vi "WM_CAP - Get Camera Name.vi"(11 "error in (no error)":errorcluster) -> (6 "FriendlyName":string, 8 "Connected?":bool, 15 "error out":errorcluster)   [LabVIEW 2022 SP3]
uses:
  <vilib>/registry/registry.llb/Registry RtKey.ctl
  <vilib>/registry/registry.llb/Read Registry Value Simple STR.vi
  <vilib>/registry/registry.llb/Read Registry Value Simple U32.vi
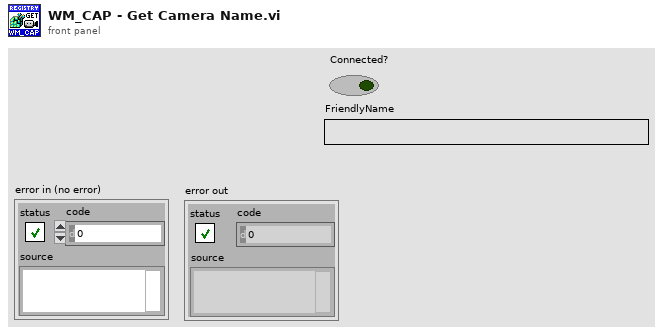
[diagram p1: front panel]
types:
  T1 = typedef "Registry RtKey.ctl" = enum32{"HKEY_CLASSES_ROOT", "HKEY_CURRENT_USER", "HKEY_LOCAL_MACHINE", "HKEY_USERS", "HKEY_PERFORMANCE_DATA", "HKEY_CURRENT_CONFIG", "HKEY_DYN_DATA"}
  T2 = typedef "Registry refnum.ctl" = refnum<k1>
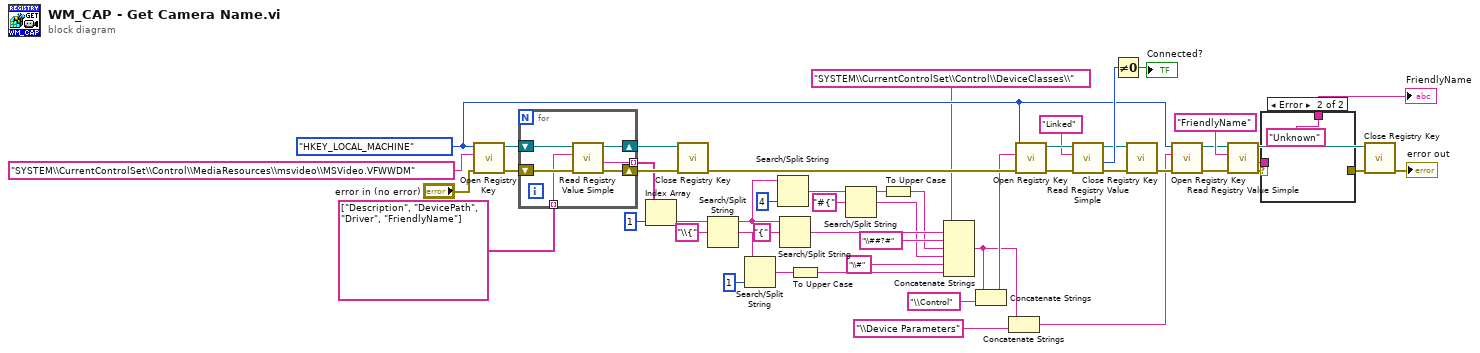
[diagram p0: block diagram]
diagram:
  w10 = Registry_RtKey."HKEY_LOCAL_MACHINE" ("root key (HKEY_LOCAL_MACHINE)")
  n1 = call <vilib>:"Open Registry Key.vi"("error in (no error)"="error in (no error)", "subkey"="SYSTEM\\CurrentControlSet\\Control\\MediaResources\\msvideo\\MSVideo.VFWWDM", "root key (HKEY_LOCAL_MACHINE)"=w10) -> ("error out"=w46:errorcluster, "refnum out"=w47:T2)  [unwired: 7 in]
  n2 = for {
    shift-right: [w55] -> w50
    shift-left: w47 -> [w57]
    shift-right: [w54] -> w49
    shift-left: w46 -> [w56]
    tunnel: string[] ["Description", "DevicePath", "Driver", "FriendlyName"] -> [w53] mode=indexing
    tunnel: [w52] -> w45 mode=indexing
    n3 = call-poly <vilib>:"Read Registry Value Simple.vi"("error in (no error)"=w56, "value"=w53, "refnum"=w57) -> ("error out"=w54:errorcluster, "String/Binary data"=w52:string, "refnum out"=w55:T2)  [unwired: 3 in, 1 out]
  }
  n4 = Index Array(array=w45, index=1) -> (element=w38:string)
  n5 = call <vilib>:"Close Registry Key.vi"("error in (no error)"=w49, "refnum"=w50) -> ("error out"=w39:errorcluster)  [unwired: 5 in]
  n6 = Search/Split String(string=w38, search string/char (-)="\\{") -> (substring before match=w35:string, match + rest of string=w41:string)  [unwired: 1 in, 1 out]
  n7 = Search/Split String(string=w41, offset (0)=1) -> (match + rest of string=w33:string)  [unwired: 1 in, 2 out]
  n8 = Search/Split String(string=w35, offset (0)=4) -> (match + rest of string=w27:string)  [unwired: 1 in, 2 out]
  n9 = Search/Split String(string=w35, search string/char (-)="{") -> (match + rest of string=w37:string)  [unwired: 1 in, 2 out]
  n10 = To Upper Case(1:w33) -> (0:w31:string)
  n11 = Search/Split String(string=w27, search string/char (-)="#{") -> (substring before match=w25:string, match + rest of string=w23:string)  [unwired: 1 in, 1 out]
  n12 = To Upper Case(1:w25) -> (0:w24:string)
  n13 = Concatenate Strings("SYSTEM\\CurrentControlSet\\Control\\DeviceClasses\\" ("subkey"), w37, "\\##?#" ("string"), w24, w23, "\\#" ("string"), w31) -> (w18:string)
  n14 = Concatenate Strings(w18, "\\Control" ("string")) -> (w19:string)
  n15 = Concatenate Strings(w18, "\\Device Parameters" ("string")) -> (w8:string)
  n16 = call <vilib>:"Open Registry Key.vi"("error in (no error)"=w39, "subkey"=w19, "root key (HKEY_LOCAL_MACHINE)"=w10) -> ("error out"=w29:errorcluster, "refnum out"=w30:T2)  [unwired: 7 in]
  n17 = call-poly <vilib>:"Read Registry Value Simple.vi"("error in (no error)"=w29, "value"="Linked", "refnum"=w30) -> ("error out"=w13:errorcluster, "DWORD data"=w22:u32, "refnum out"=w14:T2)  [unwired: 3 in, 1 out]
  n18 = Not Equal To 0?(x=w22) -> (x != 0?=→"Connected?":bool)
  n19 = call <vilib>:"Close Registry Key.vi"("error in (no error)"=w13, "refnum"=w14) -> ("error out"=w12:errorcluster)  [unwired: 5 in]
  n20 = call <vilib>:"Open Registry Key.vi"("error in (no error)"=w12, "subkey"=w8, "root key (HKEY_LOCAL_MACHINE)"=w10) -> ("error out"=w1:errorcluster, "refnum out"=w11:T2)  [unwired: 7 in]
  n21 = call-poly <vilib>:"Read Registry Value Simple.vi"("error in (no error)"=w1, "value"="FriendlyName", "refnum"=w11) -> ("error out"=w5:errorcluster, "String/Binary data"=w3:string, "refnum out"=w16:T2)  [unwired: 3 in, 1 out]
  n22 = case shown="Error" w5 {
    selector: w5 -> [w58 _]
    tunnel: [w59 "Unknown" ("String/Binary data")] -> w4
    tunnel: w3 -> [w59 _]
    tunnel: [w58 _] -> w2
    frame No Error {
    }
    frame Error {
    }
  }
  "FriendlyName" <- w4
  n23 = call <vilib>:"Close Registry Key.vi"("error in (no error)"=w2, "refnum"=w16) -> ("error out"=→"error out":errorcluster)  [unwired: 5 in]
